vi "GetInterfaceDetails.vi"(8 "error in":errorcluster, 11 "Path/ProjectItem":variant) -> (0 "error out":errorcluster)   [LabVIEW 2020, in "InterfaceLibrary.lvlib"]
uses:
  <resource>/Framework/Providers/Open_GDS/ClassProviders/Common/InterfaceLibrary/InterfaceLibrary.lvlib
  <resource>/Framework/Providers/Open_GDS/ClassProviders/Common/InterfaceLibrary/InterfaceInfo.ctl
  <resource>/Framework/Providers/Open_GDS/ClassProviders/Common/LvClass_class/GDSLvClass_ClassMethodInfo.ctl
panel:
  out "InterfaceInfo":T1
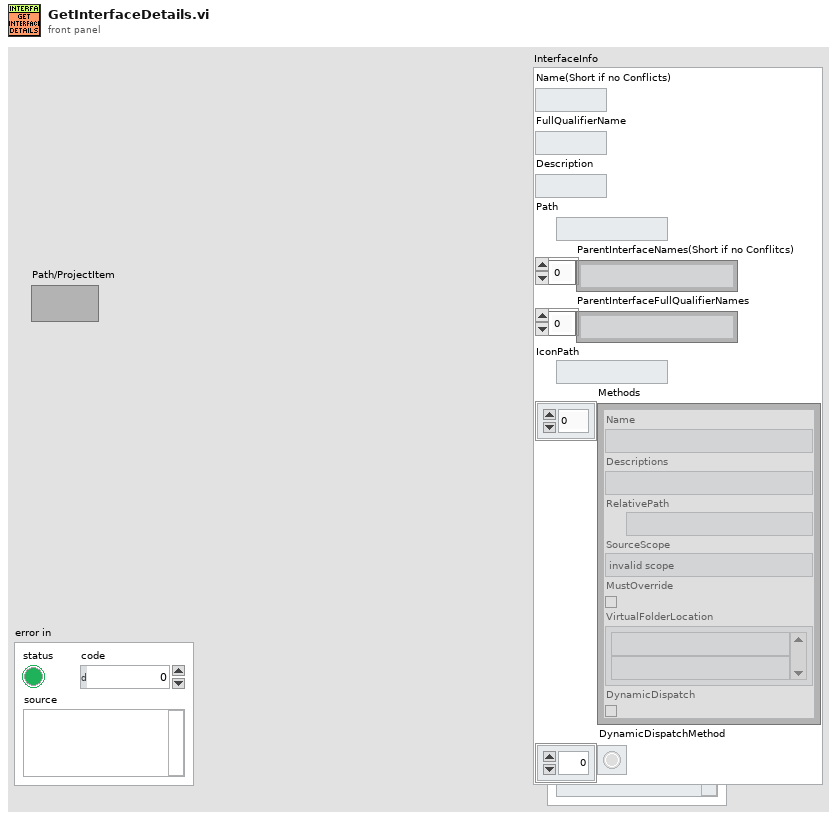
[diagram p1: front panel]
types:
  T1 = typedef "InterfaceLibrary.lvlib/InterfaceInfo.ctl" = cluster{"Name(Short if no Conflicts)":string, "FullQualifierName":string, "Description":string, "Path":path, "ParentInterfaceNames(Short if no Conflitcs)":string[], "ParentInterfaceFullQualifierNames":string[], "IconPath":path, "Methods":T2[], "DynamicDispatchMethod":bool[]}
  T2 = typedef "GDSLvClass_ClassMethodInfo.ctl" = cluster{"Name":string, "Descriptions":string, "RelativePath":path, "SourceScope":enum32{"invalid scope", "public", "private", "protected", "community"}, "MustOverride":bool, "VirtualFolderLocation":string[], "DynamicDispatch":bool}
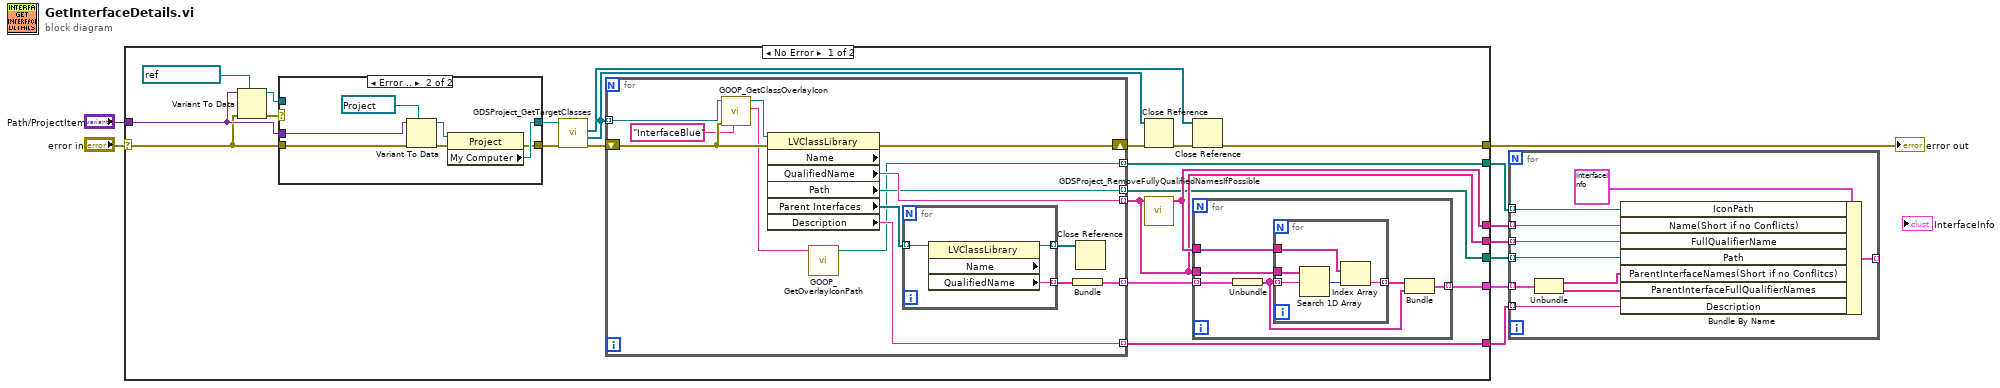
[diagram p0: block diagram]
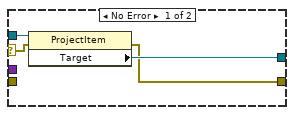
[diagram p2: hidden frame]
diagram:
  n1 = case shown="No Error" "error in" {
    selector: "error in" -> [w25 w69]
    tunnel: "Path/ProjectItem" -> [w26 _]
    tunnel: [w11 w69] -> w7
    tunnel: [w19 _] -> w5
    tunnel: [w18 _] -> w2
    tunnel: [w17 _] -> w4
    tunnel: [w16 _] -> w3
    tunnel: [w15 _] -> w1
    tunnel: [w14 _] -> w6
    frame No Error {
      n2 = Variant To Data(error in=w25, type=refnum<vi> refnum ("ProjectItem"), Variant=w26) -> (data=w28:refnum<vi>, error out=w27:errorcluster)
      n3 = case shown="Error .." w27 {
        selector: w27 -> [w58 _]
        tunnel: w28 -> [w61 _]
        tunnel: [w60 w63] -> w24
        tunnel: [w59 w62] -> w23
        tunnel: w26 -> [_ w67]
        tunnel: w25 -> [_ w66]
        frame No Error {
          n4 = property class="ProjectItem"(reference=w61, error in=w58) -> (error out=w59:errorcluster, "Target"=w60:refnum<vi>)  [unwired: 1 out]
        }
        frame Error {
          n5 = Variant To Data(error in=w66, type=refnum<vi> refnum ("ProjectItem"), Variant=w67) -> (data=w65:refnum<vi>, error out=w64:errorcluster)
          n6 = property class="Project"(reference=w65, error in=w64) -> (error out=w62:errorcluster, "My Computer"=w63:refnum<vi>)  [unwired: 1 out]
        }
      }
      n7 = call <resource>:"GDSProject_GetTargetClasses.vi"("error in (no error)"=w23, "TargetItem in"=w24) -> ("error out"=w22:errorcluster, "LvInterfaces"=w13:refnum<vi>[], "LvClasses"=w10:refnum<vi>[])  [unwired: 6 in, 1 out]
      n8 = for {
        tunnel: w13 -> [w47] mode=indexing
        tunnel: [w54] -> w17 mode=indexing
        shift-right: [w53] -> w21
        shift-left: w22 -> [w45]
        tunnel: [w50] -> w20 mode=indexing
        tunnel: [w49] -> w16 mode=indexing
        tunnel: [w48] -> w15 mode=indexing
        tunnel: [w43] -> w14 mode=indexing
        n9 = call <resource>:"GOOP_GetClassOverlayIcon.vi"("DefaultIconName(BlueFull)"="InterfaceBlue", "error in (no error)"=w45, "LVClassLibrary in"=w47) -> ("IconName"=w44:string, "LVClassLibrary out"=w46:refnum<vi>)  [unwired: 6 in, 1 out]
        n10 = property class="LVClassLibrary" props=["Name", "QualifiedName", "Path", "Parent Interfaces", "Description"](reference=w46, error in=w45) -> (error out=w53:errorcluster, "QualifiedName"=w54:string, "Path"=w49:path, "Parent Interfaces"=w52:refnum<vi>[], "Description"=w48:string)  [unwired: 2 out]
        n11 = call <resource>:"GOOP_GetOverlayIconPath.vi"("IconName(NoPngExtension)"=w44) -> ("IconPath"=w43:path)  [unwired: 10 in]
        n12 = for {
          tunnel: w52 -> [w57] mode=indexing
          tunnel: [w56] -> w51 mode=indexing
          tunnel: [w55] -> w41 mode=indexing
          n13 = property class="LVClassLibrary" props=["Name", "QualifiedName"](reference=w57) -> (reference out=w55:refnum<vi>, "QualifiedName"=w56:string)  [unwired: 1 in, 2 out]
        }
        n14 = Bundle(w51) -> (w50:cluster{string[]})  [unwired: 1 in]
        n15 = Close Reference(reference=w41) -> ()  [unwired: 1 in, 1 out]
      }
      n16 = Close Reference(reference=w13, error in (no error)=w21) -> (error out=w12:errorcluster)
      n17 = call <resource>:"GDSProject_RemoveFullyQualifiedNamesIfPossible.vi"("ItemnamesIn"=w17) -> ("ItemnamesOut"=w19:string[])  [unwired: 10 in]
      n18 = Close Reference(reference=w10, error in (no error)=w12) -> (error out=w11:errorcluster)
      n19 = for {
        tunnel: w20 -> [w35] mode=indexing
        tunnel: w17 -> [w34]
        tunnel: w19 -> [w33]
        tunnel: [w31] -> w18 mode=indexing
        n20 = Unbundle(w35) -> (w30:string[])
        n21 = for {
          tunnel: w30 -> [w40] mode=indexing
          tunnel: w34 -> [w39]
          tunnel: w33 -> [w37]
          tunnel: [w36] -> w32 mode=indexing
          n22 = Search 1D Array(1D array=w39, element=w40) -> (index of element=w38:i32)  [unwired: 1 in]
          n23 = Index Array(array=w37, index=w38) -> (element=w36:string)
        }
        n24 = Bundle(w32, w30) -> (w31:cluster{string[], string[]})  [unwired: 1 in]
      }
    }
    frame Error {
    }
  }
  "error out" <- w7
  n25 = for {
    tunnel: w6 -> [w79] mode=indexing
    tunnel: w5 -> [w78] mode=indexing
    tunnel: w4 -> [w77] mode=indexing
    tunnel: w3 -> [w76] mode=indexing
    tunnel: w2 -> [w75] mode=indexing
    tunnel: w1 -> [w72] mode=indexing
    tunnel: [w70] -> _ mode=indexing
    n26 = Unbundle(w75) -> (w74:string[], w73:string[])
    n27 = Bundle By Name(cluster=T1 {"Name(Short if no Conflicts)"="", "FullQualifierName"="", "Description"="", "Path"=path "", "ParentInterfaceNames(Short if no Conflitcs)"=[], "ParentInterfaceFullQualifierNames"=[], "IconPath"=path "", "Methods"=[], "DynamicDispatchMethod"=[]} ("InterfaceInfo"), "IconPath"=w79, "Name(Short if no Conflicts)"=w78, "FullQualifierName"=w77, "Path"=w76, "ParentInterfaceNames(Short if no Conflitcs)"=w74, "ParentInterfaceFullQualifierNames"=w73, "Description"=w72) -> (w70:T1)
  }
